vi "4461 - AI AND AI - Read AND Write.vi"(4 "Reset":bool, 6 "AO Array":waveform(dbl)[](array[waveform]), 8 "error in (no error)":errorcluster, 9 "sampling info":cluster{"Fs":dbl, "#s":dbl}={"Fs"=1000.0, "#s"=1000.0} {"Fs" format="%.2p"}, 10 "AO Task":refnum<k21>[](array[refnum]), 11 "AI task":refnum<k21>[](array[refnum])=["", ""]) -> (0 "error out":errorcluster, 3 "Input Signals":waveform(dbl)[](array[waveform]))   [LabVIEW 2013]
uses:
  <vilib>/DAQmx/write.llb/DAQmx Write (Analog 1D Wfm NChan NSamp).vi
  <vilib>/DAQmx/read.llb/DAQmx Read (Analog 1D Wfm NChan NSamp).vi
  <vilib>/DAQmx/miscellaneous.llb/DAQmx Fill In Error Info.vi
  <resource>/objmgr/daqmx.rc
panel:
  out "Numeric":i32
  out "AvailSampPerChan 4":u32
  out "AvailSampPerChan 3":u32
  out "AvailSampPerChan 2":u32
  out "AvailSampPerChan 1":u32
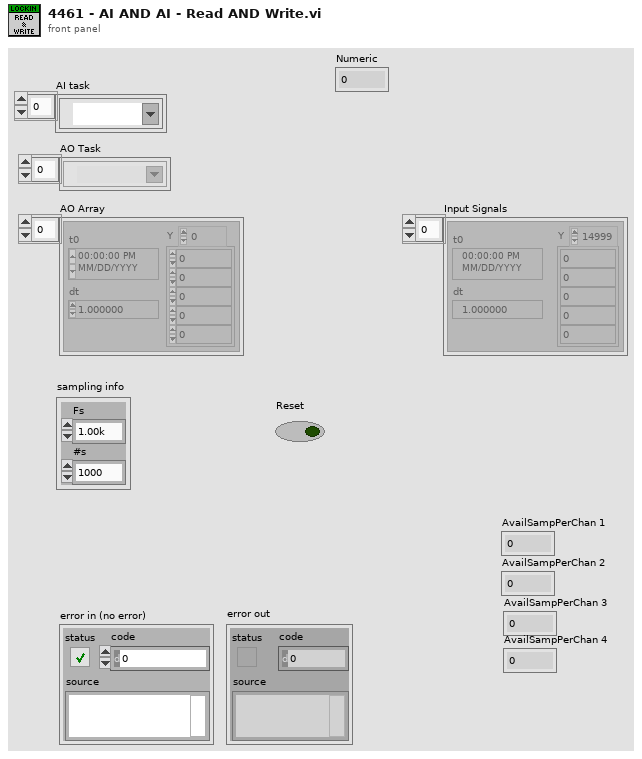
[diagram p1: front panel]
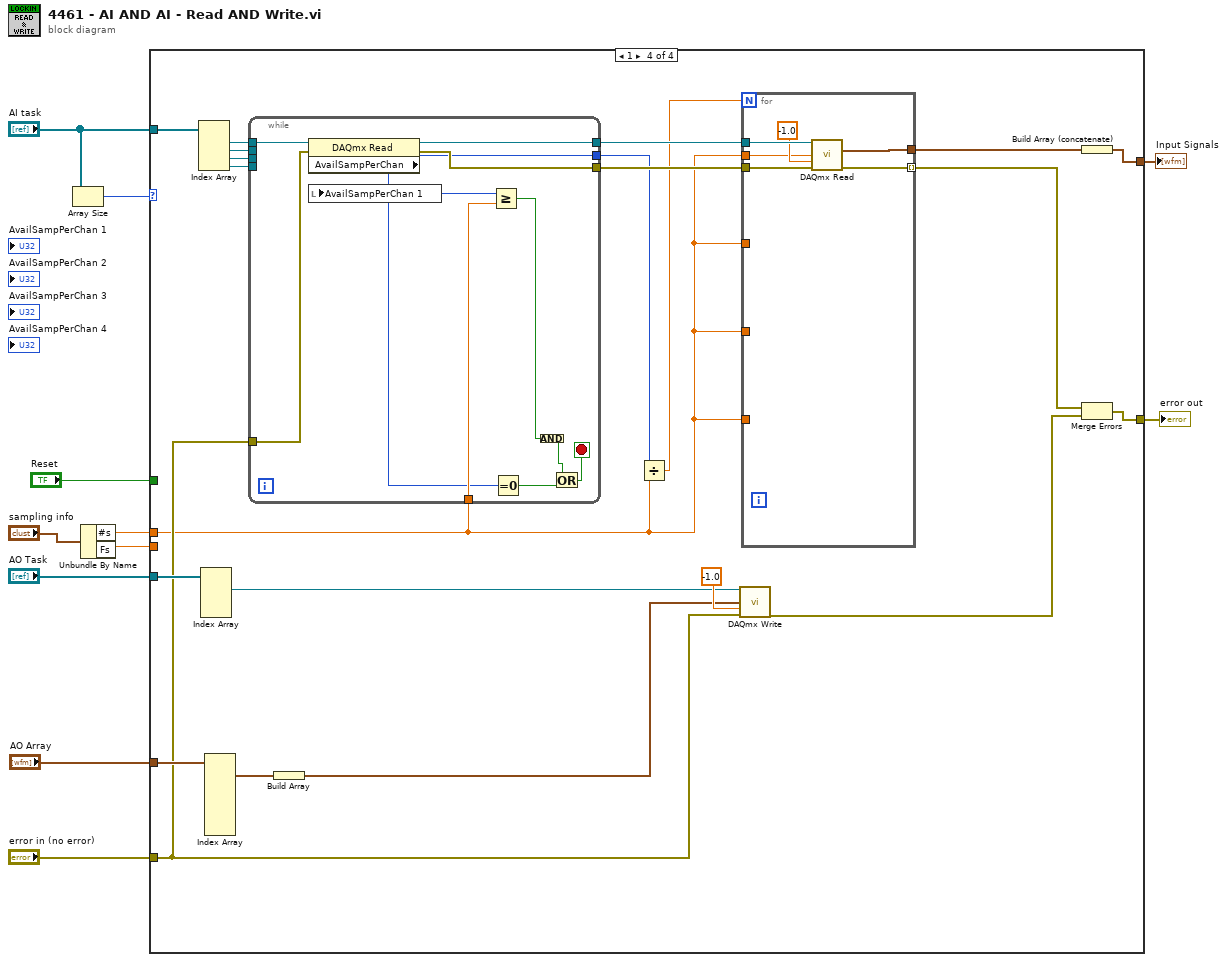
[diagram p0: block diagram]
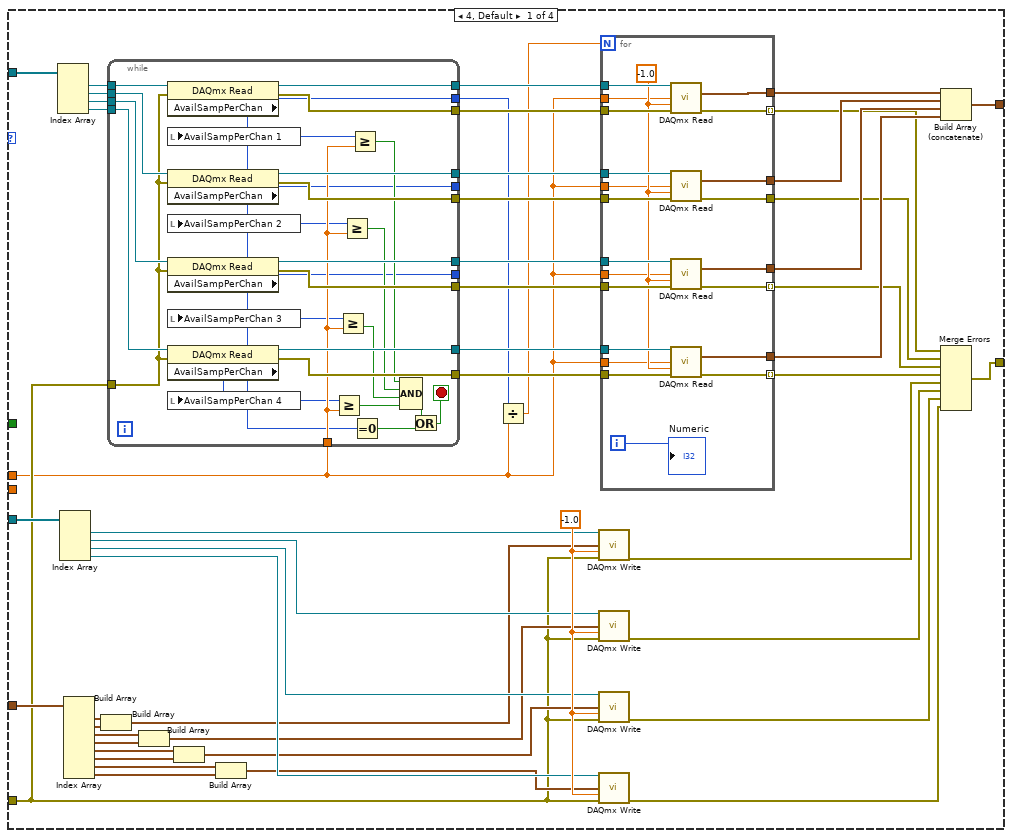
[diagram p2: hidden frame]
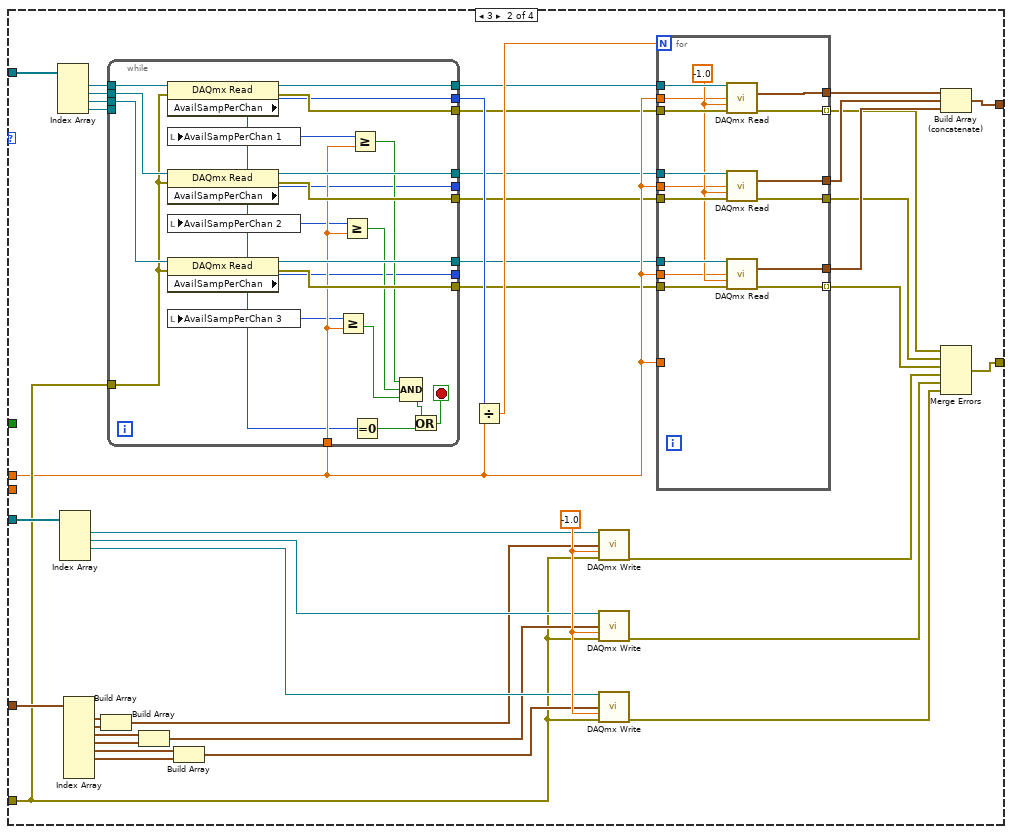
[diagram p3: hidden frame]
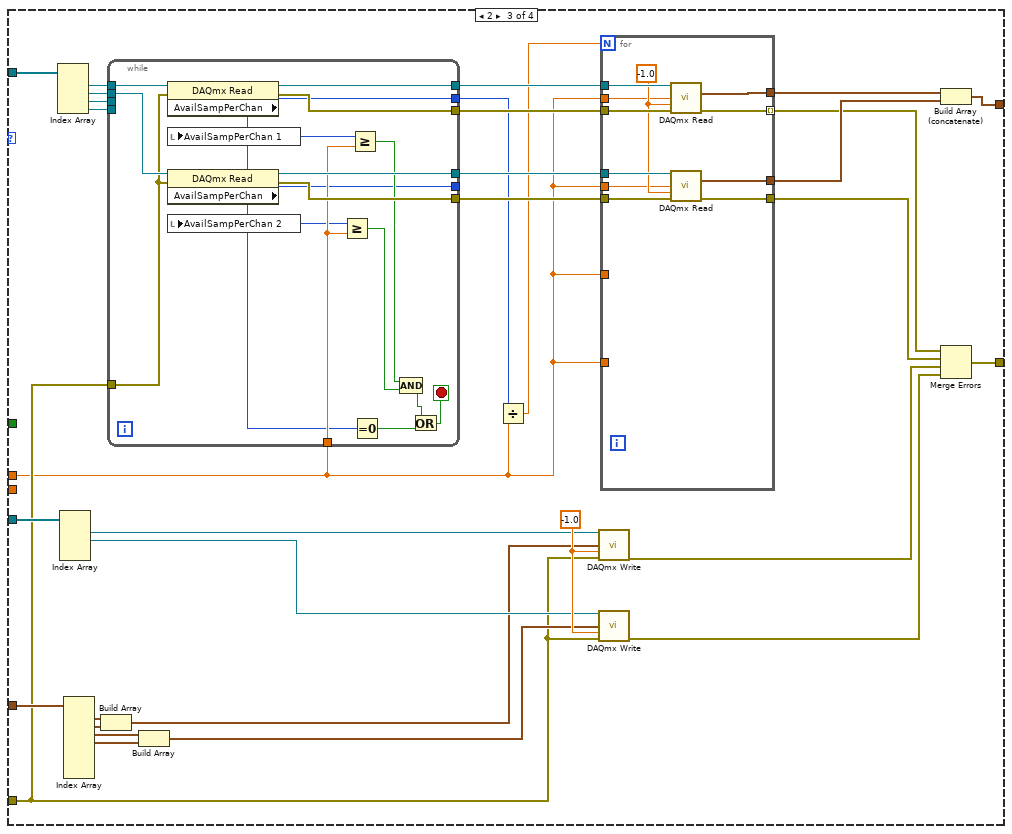
[diagram p4: hidden frame]
diagram:
  n1 = Array Size(array="AI task") -> (size(s)=w8:i32)
  n2 = Unbundle By Name("sampling info") -> ("#s"=w7:dbl, "Fs"=w2:dbl)
  n3 = case shown="1" w8 {
    tunnel: "AI task" -> [w61 w149 w217 w265]
    tunnel: [w13 w116 w187 w245] -> w3
    tunnel: "error in (no error)" -> [w28 w128 w196 w251]
    tunnel: [w60 w148 w216 w264] -> w9
    tunnel: w7 -> [w14 w117 w188 w246]
    tunnel: "AO Task" -> [w47 w143 w207 w257]
    tunnel: "AO Array" -> [w38 w136 w202 w255]
    tunnel: w2 -> [_ _ _ _]
    tunnel: "Reset" -> [_ _ _ _]
    frame 4, Default {
      w37 = -1.0 ("timeout")
      n4 = Index Array(array=w61) -> (element #1=w56:refnum<k21>, element #2=w57:refnum<k21>, element #3=w58:refnum<k21>, element #4=w59:refnum<k21>)  [unwired: 4 in]
      n5 = Index Array(array=w47) -> (element #1=w36:refnum<k21>, element #2=w35:refnum<k21>, element #3=w34:refnum<k21>, element #4=w33:refnum<k21>)  [unwired: 4 in]
      n6 = Index Array(array=w38) -> (element #1=w39:waveform(dbl), element #2=w40:waveform(dbl), element #3=w41:waveform(dbl), element #4=w42:waveform(dbl), element #5=w43:waveform(dbl), element #6=w44:waveform(dbl), element #7=w45:waveform(dbl), element #8=w46:waveform(dbl))  [unwired: 8 in]
      n7 = Build Array(w39, w40) -> (w32:waveform(dbl)[])
      n8 = while {
        tunnel: w59 -> [w108]
        tunnel: w58 -> [w107]
        tunnel: w57 -> [w106]
        tunnel: w56 -> [w105]
        tunnel: [w104] -> w55
        tunnel: [w103] -> w54
        tunnel: [w102] -> w53
        tunnel: [w101] -> w52
        tunnel: w28 -> [w96]
        tunnel: [w100] -> w51
        tunnel: [w99] -> w50
        tunnel: [w98] -> w49
        tunnel: [w97] -> w48
        tunnel: w14 -> [w90]
        tunnel: [w84] -> w12
        tunnel: [w86] -> _
        tunnel: [w85] -> _
        stop <- w88 stop-if-true
        n9 = property class="DAQmx Read"(reference=w105, error in=w96) -> (reference out=w104:refnum<k21>, error out=w100:errorcluster, "AvailSampPerChan"=w84:u32)
        n10 = local write "AvailSampPerChan 1"(w84) -> ()
        n11 = property class="DAQmx Read"(reference=w106, error in=w96) -> (reference out=w103:refnum<k21>, error out=w99:errorcluster, "AvailSampPerChan"=w85:u32)
        n12 = local write "AvailSampPerChan 2"(w85) -> ()
        n13 = property class="DAQmx Read"(reference=w107, error in=w96) -> (reference out=w102:refnum<k21>, error out=w98:errorcluster, "AvailSampPerChan"=w86:u32)
        n14 = local write "AvailSampPerChan 3"(w86) -> ()
        n15 = property class="DAQmx Read"(reference=w108, error in=w96) -> (reference out=w101:refnum<k21>, error out=w97:errorcluster, "AvailSampPerChan"=w87:u32)
        n16 = local write "AvailSampPerChan 4"(w87) -> ()
        n17 = Greater Or Equal?(x=w87, y=w90) -> (x >= y?=w95:bool)
        n18 = Greater Or Equal?(x=w86, y=w90) -> (x >= y?=w94:bool)
        n19 = Greater Or Equal?(x=w85, y=w90) -> (x >= y?=w93:bool)
        n20 = Greater Or Equal?(x=w84, y=w90) -> (x >= y?=w92:bool)
        n21 = Equal To 0?(x=w84) -> (x = 0?=w89:bool)
        n22 = Compound Arithmetic op=AND(w92, w93, w94, w95) -> (w91:bool)
        n23 = Or(x=w91, y=w89) -> (x .or. y?=w88:bool)
      }
      n24 = Build Array(w41, w42) -> (w31:waveform(dbl)[])
      n25 = Build Array(w43, w44) -> (w30:waveform(dbl)[])
      n26 = Build Array(w45, w46) -> (w29:waveform(dbl)[])
      n27 = Divide(x=w12, y=w14) -> (x/y=w15:dbl)
      n28 = call-poly <vilib>:"DAQmx Write.vi"("task/channels in"=w36, "data"=w32, "timeout"=w37, "error in"=w28) -> ("error out"=w27:errorcluster)  [unwired: 9 in, 2 out]
      n29 = call-poly <vilib>:"DAQmx Write.vi"("task/channels in"=w35, "data"=w31, "timeout"=w37, "error in"=w28) -> ("error out"=w26:errorcluster)  [unwired: 9 in, 2 out]
      n30 = call-poly <vilib>:"DAQmx Write.vi"("task/channels in"=w34, "data"=w30, "timeout"=w37, "error in"=w28) -> ("error out"=w25:errorcluster)  [unwired: 9 in, 2 out]
      n31 = call-poly <vilib>:"DAQmx Write.vi"("task/channels in"=w33, "data"=w29, "timeout"=w37, "error in"=w28) -> ("error out"=w24:errorcluster)  [unwired: 9 in, 2 out]
      n32 = for {
        N: w15 -> [_]
        tunnel: w55 -> [w83]
        tunnel: w54 -> [w82]
        tunnel: w53 -> [w81]
        tunnel: w52 -> [w80]
        tunnel: w51 -> [w79]
        tunnel: w50 -> [w78]
        tunnel: w49 -> [w77]
        tunnel: w48 -> [w76]
        tunnel: [w74] -> w23
        tunnel: [w73] -> w22
        tunnel: [w72] -> w21
        tunnel: [w71] -> w20
        tunnel: w14 -> [w70]
        tunnel: w14 -> [w69]
        tunnel: w14 -> [w68]
        tunnel: w14 -> [w67]
        tunnel: [w66] -> w19 mode=indexing
        tunnel: [w65] -> w18
        tunnel: [w64] -> w17 mode=indexing
        tunnel: [w63] -> w16 mode=indexing
        i -> [w62]
        w75 = -1.0 ("timeout")
        n33 = call-poly <vilib>:"DAQmx Read.vi"("task/channels in"=w83, "number of samples per channel"=w69, "timeout"=w75, "error in"=w79) -> ("data"=w73:waveform(dbl)[], "error out"=w66:errorcluster)  [unwired: 9 in, 1 out]
        n34 = call-poly <vilib>:"DAQmx Read.vi"("task/channels in"=w82, "number of samples per channel"=w67, "timeout"=w75, "error in"=w78) -> ("data"=w74:waveform(dbl)[], "error out"=w65:errorcluster)  [unwired: 9 in, 1 out]
        n35 = call-poly <vilib>:"DAQmx Read.vi"("task/channels in"=w81, "number of samples per channel"=w68, "timeout"=w75, "error in"=w77) -> ("data"=w72:waveform(dbl)[], "error out"=w64:errorcluster)  [unwired: 9 in, 1 out]
        n36 = call-poly <vilib>:"DAQmx Read.vi"("task/channels in"=w80, "number of samples per channel"=w70, "timeout"=w75, "error in"=w76) -> ("data"=w71:waveform(dbl)[], "error out"=w63:errorcluster)  [unwired: 9 in, 1 out]
        "Numeric" <- w62
      }
      n37 = Build Array (concatenate)(w22, w23, w21, w20) -> (w13:waveform(dbl)[])
      n38 = Merge Errors(w19, w18, w17, w16, w27, w26, w25, w24) -> (w60:errorcluster)
    }
    frame 3 {
      w135 = -1.0 ("timeout")
      n39 = Index Array(array=w149) -> (element #1=w144:refnum<k21>, element #2=w145:refnum<k21>, element #3=w146:refnum<k21>, element #4=w147:refnum<k21>)  [unwired: 4 in]
      n40 = Index Array(array=w143) -> (element #1=w134:refnum<k21>, element #2=w133:refnum<k21>, element #3=w132:refnum<k21>)  [unwired: 4 in, 1 out]
      n41 = Index Array(array=w136) -> (element #1=w137:waveform(dbl), element #2=w138:waveform(dbl), element #3=w139:waveform(dbl), element #4=w140:waveform(dbl), element #5=w141:waveform(dbl), element #6=w142:waveform(dbl))  [unwired: 8 in, 2 out]
      n42 = Build Array(w137, w138) -> (w131:waveform(dbl)[])
      n43 = while {
        tunnel: w147 -> [_]
        tunnel: w146 -> [w185]
        tunnel: w145 -> [w184]
        tunnel: w144 -> [w183]
        tunnel: [w182] -> w109
        tunnel: [w181] -> w111
        tunnel: [w180] -> w113
        tunnel: w128 -> [w176]
        tunnel: [w179] -> w110
        tunnel: [w178] -> w112
        tunnel: [w177] -> w114
        tunnel: w117 -> [w171]
        tunnel: [w166] -> w115
        tunnel: [w168] -> _
        tunnel: [w167] -> _
        stop <- w169 stop-if-true
        n44 = property class="DAQmx Read"(reference=w183, error in=w176) -> (reference out=w182:refnum<k21>, error out=w179:errorcluster, "AvailSampPerChan"=w166:u32)
        n45 = local write "AvailSampPerChan 1"(w166) -> ()
        n46 = property class="DAQmx Read"(reference=w184, error in=w176) -> (reference out=w181:refnum<k21>, error out=w178:errorcluster, "AvailSampPerChan"=w167:u32)
        n47 = local write "AvailSampPerChan 2"(w167) -> ()
        n48 = property class="DAQmx Read"(reference=w185, error in=w176) -> (reference out=w180:refnum<k21>, error out=w177:errorcluster, "AvailSampPerChan"=w168:u32)
        n49 = local write "AvailSampPerChan 3"(w168) -> ()
        n50 = Greater Or Equal?(x=w168, y=w171) -> (x >= y?=w175:bool)
        n51 = Greater Or Equal?(x=w167, y=w171) -> (x >= y?=w174:bool)
        n52 = Greater Or Equal?(x=w166, y=w171) -> (x >= y?=w173:bool)
        n53 = Equal To 0?(x=w166) -> (x = 0?=w170:bool)
        n54 = Compound Arithmetic op=AND(w173, w174, w175) -> (w172:bool)
        n55 = Or(x=w172, y=w170) -> (x .or. y?=w169:bool)
      }
      n56 = Build Array(w139, w140) -> (w130:waveform(dbl)[])
      n57 = Build Array(w141, w142) -> (w129:waveform(dbl)[])
      n58 = Divide(x=w115, y=w117) -> (x/y=w118:dbl)
      n59 = call-poly <vilib>:"DAQmx Write.vi"("task/channels in"=w134, "data"=w131, "timeout"=w135, "error in"=w128) -> ("error out"=w127:errorcluster)  [unwired: 9 in, 2 out]
      n60 = call-poly <vilib>:"DAQmx Write.vi"("task/channels in"=w133, "data"=w130, "timeout"=w135, "error in"=w128) -> ("error out"=w126:errorcluster)  [unwired: 9 in, 2 out]
      n61 = call-poly <vilib>:"DAQmx Write.vi"("task/channels in"=w132, "data"=w129, "timeout"=w135, "error in"=w128) -> ("error out"=w125:errorcluster)  [unwired: 9 in, 2 out]
      n62 = for {
        N: w118 -> [_]
        tunnel: w109 -> [w165]
        tunnel: w111 -> [w164]
        tunnel: w113 -> [w163]
        tunnel: w110 -> [w162]
        tunnel: w112 -> [w161]
        tunnel: w114 -> [w160]
        tunnel: [w158] -> w124
        tunnel: [w157] -> w123
        tunnel: [w156] -> w122
        tunnel: w117 -> [_]
        tunnel: w117 -> [w155]
        tunnel: w117 -> [w154]
        tunnel: w117 -> [w153]
        tunnel: [w152] -> w121 mode=indexing
        tunnel: [w151] -> w120
        tunnel: [w150] -> w119 mode=indexing
        w159 = -1.0 ("timeout")
        n63 = call-poly <vilib>:"DAQmx Read.vi"("task/channels in"=w165, "number of samples per channel"=w155, "timeout"=w159, "error in"=w162) -> ("data"=w157:waveform(dbl)[], "error out"=w152:errorcluster)  [unwired: 9 in, 1 out]
        n64 = call-poly <vilib>:"DAQmx Read.vi"("task/channels in"=w164, "number of samples per channel"=w153, "timeout"=w159, "error in"=w161) -> ("data"=w158:waveform(dbl)[], "error out"=w151:errorcluster)  [unwired: 9 in, 1 out]
        n65 = call-poly <vilib>:"DAQmx Read.vi"("task/channels in"=w163, "number of samples per channel"=w154, "timeout"=w159, "error in"=w160) -> ("data"=w156:waveform(dbl)[], "error out"=w150:errorcluster)  [unwired: 9 in, 1 out]
      }
      n66 = Build Array (concatenate)(w123, w124, w122) -> (w116:waveform(dbl)[])
      n67 = Merge Errors(w121, w120, w119, w127, w126, w125) -> (w148:errorcluster)
    }
    frame 2 {
      w201 = -1.0 ("timeout")
      n68 = Index Array(array=w217) -> (element #1=w212:refnum<k21>, element #2=w213:refnum<k21>, element #3=w214:refnum<k21>, element #4=w215:refnum<k21>)  [unwired: 4 in]
      n69 = Index Array(array=w207) -> (element #1=w200:refnum<k21>, element #2=w199:refnum<k21>)  [unwired: 4 in, 2 out]
      n70 = Index Array(array=w202) -> (element #1=w203:waveform(dbl), element #2=w204:waveform(dbl), element #3=w205:waveform(dbl), element #4=w206:waveform(dbl))  [unwired: 8 in, 4 out]
      n71 = Build Array(w203, w204) -> (w198:waveform(dbl)[])
      n72 = while {
        tunnel: w215 -> [_]
        tunnel: w214 -> [_]
        tunnel: w213 -> [w243]
        tunnel: w212 -> [w242]
        tunnel: [w241] -> w211
        tunnel: [w240] -> w210
        tunnel: w196 -> [w237]
        tunnel: [w239] -> w209
        tunnel: [w238] -> w208
        tunnel: w188 -> [w233]
        tunnel: [w229] -> w186
        tunnel: [w230] -> _
        stop <- w231 stop-if-true
        n73 = property class="DAQmx Read"(reference=w242, error in=w237) -> (reference out=w241:refnum<k21>, error out=w239:errorcluster, "AvailSampPerChan"=w229:u32)
        n74 = local write "AvailSampPerChan 1"(w229) -> ()
        n75 = property class="DAQmx Read"(reference=w243, error in=w237) -> (reference out=w240:refnum<k21>, error out=w238:errorcluster, "AvailSampPerChan"=w230:u32)
        n76 = local write "AvailSampPerChan 2"(w230) -> ()
        n77 = Greater Or Equal?(x=w230, y=w233) -> (x >= y?=w236:bool)
        n78 = Greater Or Equal?(x=w229, y=w233) -> (x >= y?=w235:bool)
        n79 = Equal To 0?(x=w229) -> (x = 0?=w232:bool)
        n80 = Compound Arithmetic op=AND(w235, w236) -> (w234:bool)
        n81 = Or(x=w234, y=w232) -> (x .or. y?=w231:bool)
      }
      n82 = Build Array(w205, w206) -> (w197:waveform(dbl)[])
      n83 = Divide(x=w186, y=w188) -> (x/y=w189:dbl)
      n84 = call-poly <vilib>:"DAQmx Write.vi"("task/channels in"=w200, "data"=w198, "timeout"=w201, "error in"=w196) -> ("error out"=w195:errorcluster)  [unwired: 9 in, 2 out]
      n85 = call-poly <vilib>:"DAQmx Write.vi"("task/channels in"=w199, "data"=w197, "timeout"=w201, "error in"=w196) -> ("error out"=w194:errorcluster)  [unwired: 9 in, 2 out]
      n86 = for {
        N: w189 -> [_]
        tunnel: w211 -> [w228]
        tunnel: w210 -> [w227]
        tunnel: w209 -> [w226]
        tunnel: w208 -> [w225]
        tunnel: [w223] -> w193
        tunnel: [w222] -> w192
        tunnel: w188 -> [_]
        tunnel: w188 -> [w221]
        tunnel: w188 -> [_]
        tunnel: w188 -> [w220]
        tunnel: [w219] -> w191 mode=indexing
        tunnel: [w218] -> w190
        w224 = -1.0 ("timeout")
        n87 = call-poly <vilib>:"DAQmx Read.vi"("task/channels in"=w228, "number of samples per channel"=w221, "timeout"=w224, "error in"=w226) -> ("data"=w222:waveform(dbl)[], "error out"=w219:errorcluster)  [unwired: 9 in, 1 out]
        n88 = call-poly <vilib>:"DAQmx Read.vi"("task/channels in"=w227, "number of samples per channel"=w220, "timeout"=w224, "error in"=w225) -> ("data"=w223:waveform(dbl)[], "error out"=w218:errorcluster)  [unwired: 9 in, 1 out]
      }
      n89 = Build Array (concatenate)(w192, w193) -> (w187:waveform(dbl)[])
      n90 = Merge Errors(w191, w190, w195, w194) -> (w216:errorcluster)
    }
    frame 1 {
      n91 = Index Array(array=w265) -> (element #1=w260:refnum<k21>, element #2=w261:refnum<k21>, element #3=w262:refnum<k21>, element #4=w263:refnum<k21>)  [unwired: 4 in]
      n92 = Index Array(array=w257) -> (element #1=w253:refnum<k21>)  [unwired: 4 in, 3 out]
      n93 = Index Array(array=w255) -> (element #1=w256:waveform(dbl))  [unwired: 8 in, 7 out]
      n94 = while {
        tunnel: w263 -> [_]
        tunnel: w262 -> [_]
        tunnel: w261 -> [_]
        tunnel: w260 -> [w281]
        tunnel: [w280] -> w259
        tunnel: w251 -> [w278]
        tunnel: [w279] -> w258
        tunnel: w246 -> [w275]
        tunnel: [w272] -> w244
        stop <- w273 stop-if-true
        n95 = property class="DAQmx Read"(reference=w281, error in=w278) -> (reference out=w280:refnum<k21>, error out=w279:errorcluster, "AvailSampPerChan"=w272:u32)
        n96 = local write "AvailSampPerChan 1"(w272) -> ()
        n97 = Greater Or Equal?(x=w272, y=w275) -> (x >= y?=w277:bool)
        n98 = Equal To 0?(x=w272) -> (x = 0?=w274:bool)
        n99 = Compound Arithmetic op=AND(w277) -> (w276:bool)
        n100 = Or(x=w276, y=w274) -> (x .or. y?=w273:bool)
      }
      n101 = Build Array(w256) -> (w252:waveform(dbl)[])
      n102 = Divide(x=w244, y=w246) -> (x/y=w247:dbl)
      n103 = call-poly <vilib>:"DAQmx Write.vi"("task/channels in"=w253, "data"=w252, "timeout"=-1.0, "error in"=w251) -> ("error out"=w250:errorcluster)  [unwired: 9 in, 2 out]
      n104 = for {
        N: w247 -> [_]
        tunnel: w259 -> [w271]
        tunnel: w258 -> [w270]
        tunnel: [w268] -> w249
        tunnel: w246 -> [_]
        tunnel: w246 -> [w267]
        tunnel: w246 -> [_]
        tunnel: w246 -> [_]
        tunnel: [w266] -> w248 mode=indexing
        n105 = call-poly <vilib>:"DAQmx Read.vi"("task/channels in"=w271, "number of samples per channel"=w267, "timeout"=-1.0, "error in"=w270) -> ("data"=w268:waveform(dbl)[], "error out"=w266:errorcluster)  [unwired: 9 in, 1 out]
      }
      n106 = Build Array (concatenate)(w249) -> (w245:waveform(dbl)[])
      n107 = Merge Errors(w248, w250) -> (w264:errorcluster)
    }
  }
  "Input Signals" <- w3
  "error out" <- w9
